vi "GoalieNormal.vi"(7 "AI Parameters":T1={"GotoKick"={"Dist do cone a frente"=0.0, "attacker farback"=1000.0, "Perto"=300.0, "min dist to kick"=0.0, "kick eps"=110.0, "Time to transition"=0.05}, "Attacker"={"CC chute"=0.09, "CC passe"=0.045, "Kick Force"=200.0, "D ball-robot Kick"=200.0, "D ball-robot Pass"=0.0}, "Defender"={"D max"=1700.0, "Vel p/ robô av"=1000.0, "Kick Force"=100.0, "D atk-def"=300.0, "D farback"=400.0}, "Timeout"={"Field/v in x"=6.0, "Dist Robots"=300, "Dist up in y"=300}, "Pose Striker"={"dist"=200.0, "Numeric"=-4.0, "dist 2"=200.0}, "Dist Stop"=300.0, "Distance when ball out"=200, "D central gap "=150.0} {"D central gap" format="%#_13g"; "Dist Stop" format="%#_13g"; "Pose Striker"."Numeric" format="%#_13g"; "Defender"."Kick Force" format="%#_13g"; "Defender"."Vel p/ robô av" format="%#_13g"; "Attacker"."D ball-robot Kick" format="%#_13g"; "Attacker"."Kick Force" format="%#_13g"; "Attacker"."CC passe" format="%#_13g"; "Attacker"."CC chute" format="%#_13g"; "GotoKick"."min dist to kick" format="%#_13g"; "GotoKick"."Perto" format="%#_13g"; "GotoKick"."attacker farback" format="%#_13g"; "GotoKick"."Dist do cone a frente" format="%#_13g"}, 8 "Robot":T2={"id"=0, "function"=enum."Attacker", "x"=0.0, "y"=0.0, "orientation"=0.0, "v_tangent"=0.0, "v_normal"=0.0, "v_ang"=0.0, "kick_x"=0.0, "kick_z"=0.0, "dribble"=FALSE, "Timestamp"=timestamp(0 s since 1904-01-01), "dest_x"=0.0, "dest_y"=0.0, "dest_orientation"=0.0, "estimatives"={"est_v_tangent"=0.0, "est_v_normal"=0.0, "est_vx"=0.0, "est_vy"=0.0, "Pos Robot Est"=[]}, "dest_x_kick"=0.0, "dest_y_kick"=0.0, "Gap Coord"=[], "States"=enum."GoToTangent"}, 10 "Field defense":dbl[](array[numeric]), 11 "IA Input":T5={"our_robots"=[], "enemy_robots"=[], "balls"=[], "geometry"={"line_width"=0, "field_length"=0, "field_width"=0, "boundary_width"=0, "referee_width"=0, "goal_width"=0, "goal_depth"=0, "goal_wall_width"=0, "center_circle_radius"=0, "defense_radius"=0, "defense_stretch"=0, "free_kick_from_defense_dist"=0, "penalty_spot_from_field_line_dist"=0, "penalty_line_from_spot_dist"=0}, "IA Judge"={"stage"="", "command"="", "our_goalie_id"=0.0, "enemy_goalie_id"=0.0, "command enum"=enum."Halt", "Time"=enum."Azul"}, "Received Timestamp"=timestamp(0 s since 1904-01-01), "Events"={"Touch"=FALSE, "Ball out"=FALSE, "id touch"=0.0, "Ball out of \nVision"=FALSE, "Ball inside \nGoalie area"=FALSE, "Robot not responding"=FALSE, "Robots responding status"=[1.0, 1.0, 1.0, 1.0, 1.0, 1.0], "Enemy Ball \nPossession"=FALSE, "Pass State"=FALSE, "id end of pass"=0.0, "Kick"=FALSE, "Id Possession"=0.0}}) -> (2 "output cluster":T2={"id"=0, "function"=enum."Attacker", "x"=0.0, "y"=0.0, "orientation"=0.0, "v_tangent"=0.0, "v_normal"=0.0, "v_ang"=0.0, "kick_x"=0.0, "kick_z"=0.0, "dribble"=FALSE, "Timestamp"=timestamp(0 s since 1904-01-01), "dest_x"=0.0, "dest_y"=0.0, "dest_orientation"=0.0, "estimatives"={"est_v_tangent"=0.0, "est_v_normal"=0.0, "est_vx"=0.0, "est_vy"=0.0, "Pos Robot Est"=[]}, "dest_x_kick"=0.0, "dest_y_kick"=0.0, "Gap Coord"=[], "States"=enum."GoToTangent"})   [LabVIEW 2016]
uses:
  Core/AI Input.ctl
  Core/AI Robot.ctl
  Functions Enum.ctl
  AttackerStates.ctl
  Core/AI Ball.ctl
  Core/Field Size.ctl
  Core/AI Judge.ctl
  Command Enum.ctl
  Util/Events/Events.ctl
  AI Parameters.ctl
panel:
  in  "Time kick (s)":dbl=1.0 caption="Time Target (s)"
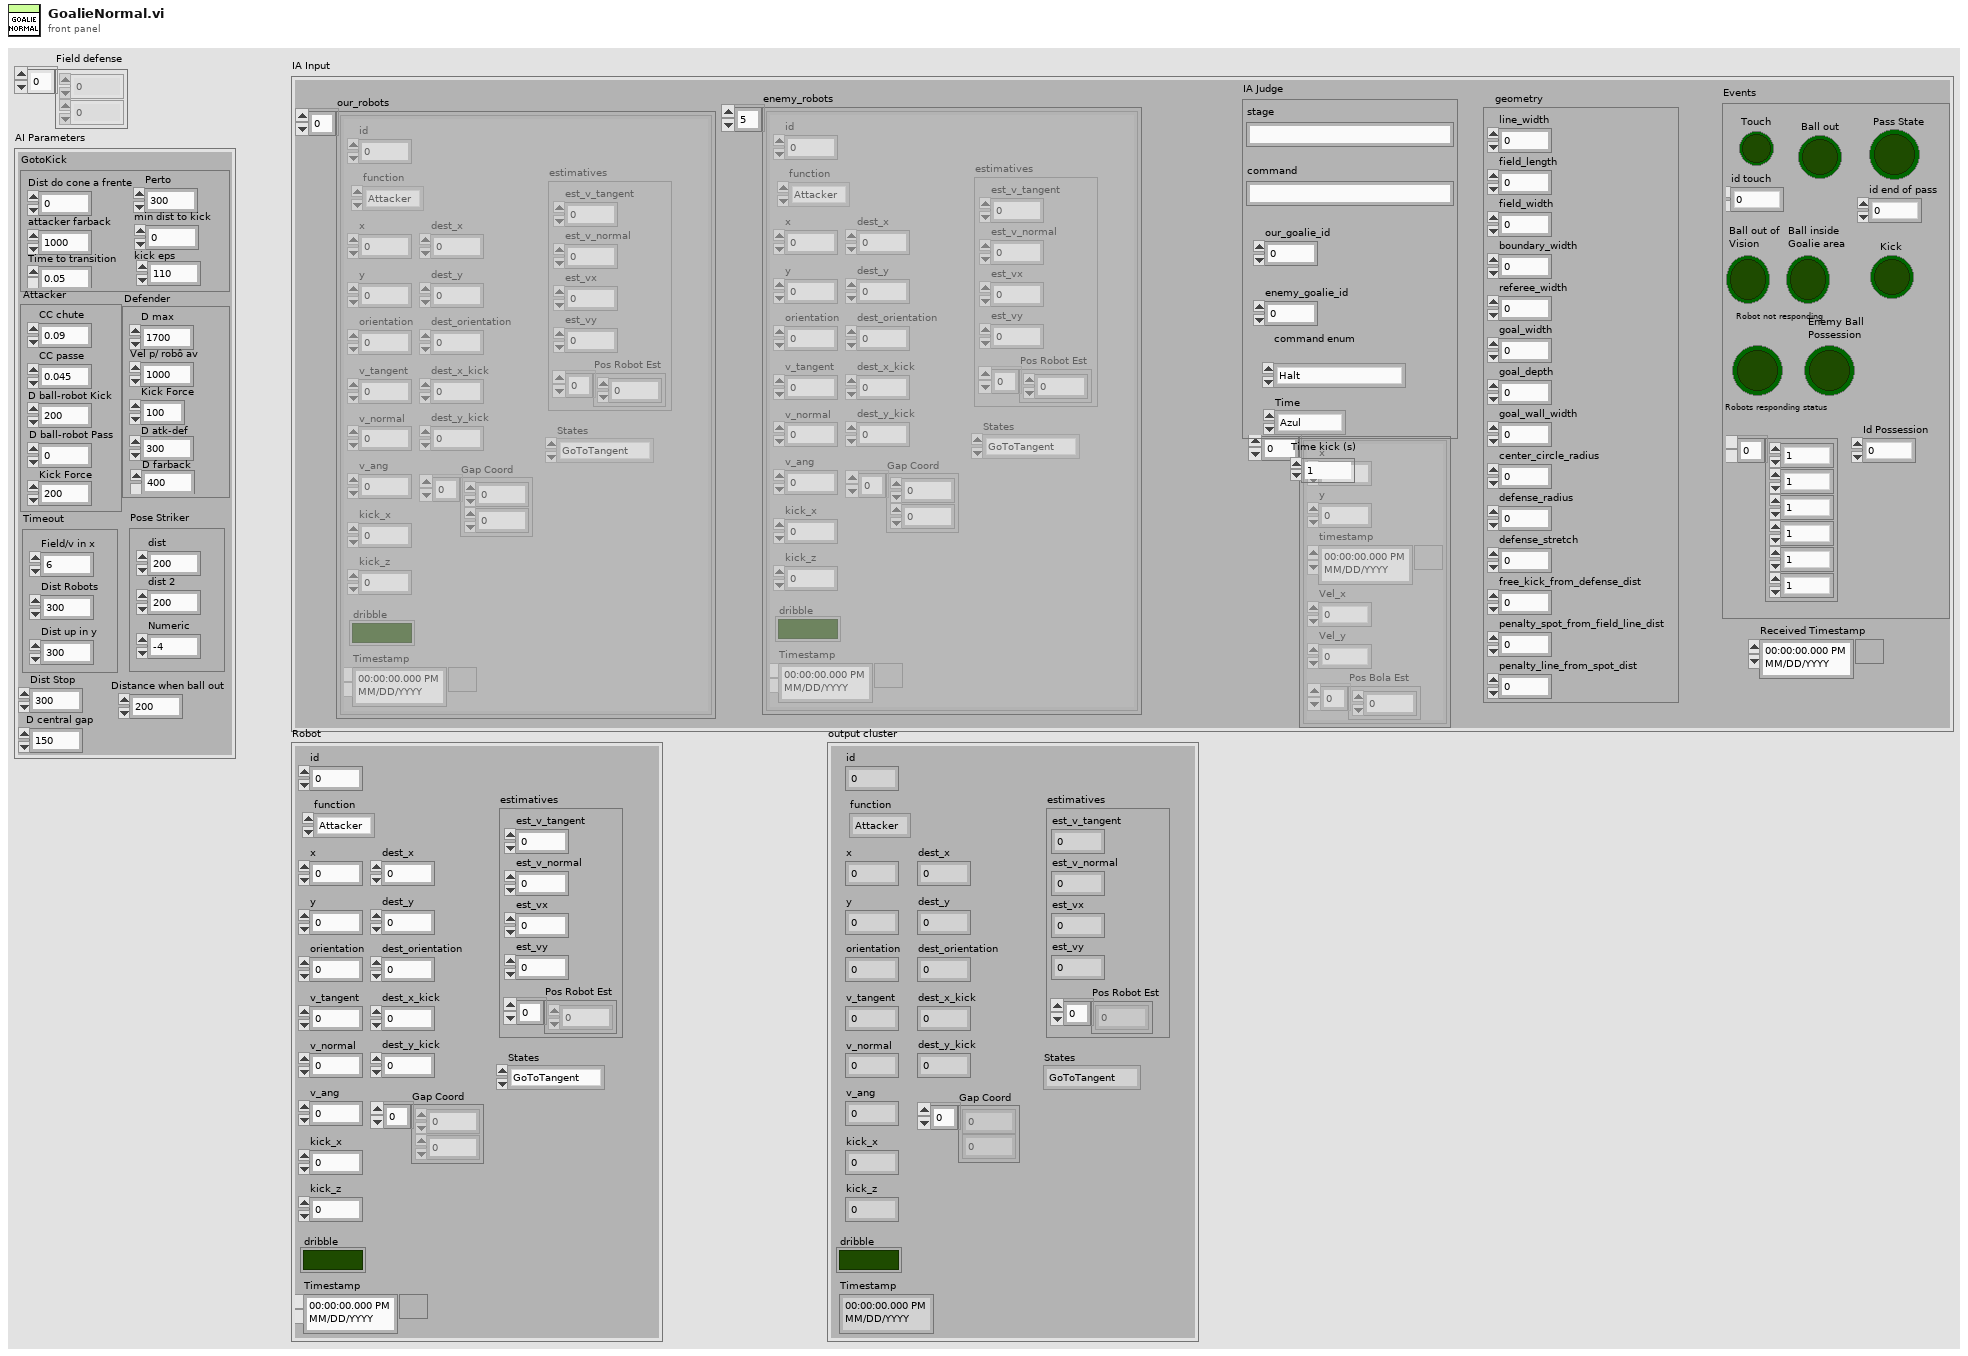
[diagram p1: front panel]
types:
  T1 = typedef "AI Parameters.ctl" = cluster{"GotoKick":cluster{"Dist do cone a frente":dbl, "attacker farback":dbl, "Perto":dbl, "min dist to kick":dbl, "kick eps":dbl, "Time to transition":dbl}, "Attacker":cluster{"CC chute":dbl, "CC passe":dbl, "Kick Force":dbl, "D ball-robot Kick":dbl, "D ball-robot Pass":dbl}, "Defender":cluster{"D max":dbl, "Vel p/ robô av":dbl, "Kick Force":dbl, "D atk-def":dbl, "D farback":dbl}, "Timeout":cluster{"Field/v in x":dbl, "Dist Robots":u32, "Dist up in y":u32}, "Pose Striker":cluster{"dist":dbl, "Numeric":dbl, "dist 2":dbl}, "Dist Stop":dbl, "Distance when ball out":i32, "D central gap ":dbl}
  T2 = typedef "AI Robot.ctl" = cluster{"id":u32, "function":T3, "x":dbl, "y":dbl, "orientation":dbl, "v_tangent":dbl, "v_normal":dbl, "v_ang":dbl, "kick_x":dbl, "kick_z":dbl, "dribble":bool, "Timestamp":timestamp, "dest_x":dbl, "dest_y":dbl, "dest_orientation":dbl, "estimatives":cluster{"est_v_tangent":dbl, "est_v_normal":dbl, "est_vx":dbl, "est_vy":dbl, "Pos Robot Est":dbl[]}, "dest_x_kick":dbl, "dest_y_kick":dbl, "Gap Coord":dbl[], "States":T4}
  T3 = typedef "Functions Enum.ctl" = enum16{"Attacker", "Goalie", "Defender", "Striker", "Goto 0", "Dummy", "Kicker", "ZigZag"}
  T4 = typedef "AttackerStates.ctl" = enum16{"Pass", "GoToTangent", "BallGetting", "GoToKick", ""}
  T5 = typedef "AI Input.ctl" = cluster{"our_robots":T2[], "enemy_robots":T2[], "balls":T6[], "geometry":T7, "IA Judge":T8, "Received Timestamp":timestamp, "Events":T10}
  T6 = typedef "AI Ball.ctl" = cluster{"x":dbl, "y":dbl, "timestamp":timestamp, "Vel_x":dbl, "Vel_y":dbl, "Pos Bola Est":dbl[]}
  T7 = typedef "Field Size.ctl" = cluster{"line_width":u32, "field_length":u32, "field_width":u32, "boundary_width":u32, "referee_width":u32, "goal_width":u32, "goal_depth":u32, "goal_wall_width":u32, "center_circle_radius":u32, "defense_radius":u32, "defense_stretch":u32, "free_kick_from_defense_dist":u32, "penalty_spot_from_field_line_dist":u32, "penalty_line_from_spot_dist":u32}
  T8 = typedef "AI Judge.ctl" = cluster{"stage":string, "command":string, "our_goalie_id":dbl, "enemy_goalie_id":dbl, "command enum":T9, "Time":enum16{"Azul", "Amarelo"}}
  T9 = typedef "Command Enum.ctl" = enum16{"Halt", "Stop", "Force Start", "PKA Normal Start", "Prepare Kickoff Ally", "PKE Normal Start", "Prepare Kickoff Enemy", "Prepare Penalty Ally", "PPA Normal Start", "Prepare Penalty Enemy", "PPE Normal Start", "Direct Free Enemy", "Direct Free Ally", "Indirect Free Enemy", "Indirect Free Ally", "Timeout Enemy", "Timeout Ally", "Goal Enemy", "Goal Ally", "Ball Placement Enemy", "Ball Placement Ally", "Normal Half Time", "Extra Time Break", "Extra Half Time", "None"}
  T10 = typedef "Events.ctl" = cluster{"Touch":bool, "Ball out":bool, "id touch":dbl, "Ball out of \nVision":bool, "Ball inside \nGoalie area":bool, "Robot not responding":bool, "Robots responding status":dbl[], "Enemy Ball \nPossession":bool, "Pass State":bool, "id end of pass":dbl, "Kick":bool, "Id Possession":dbl}
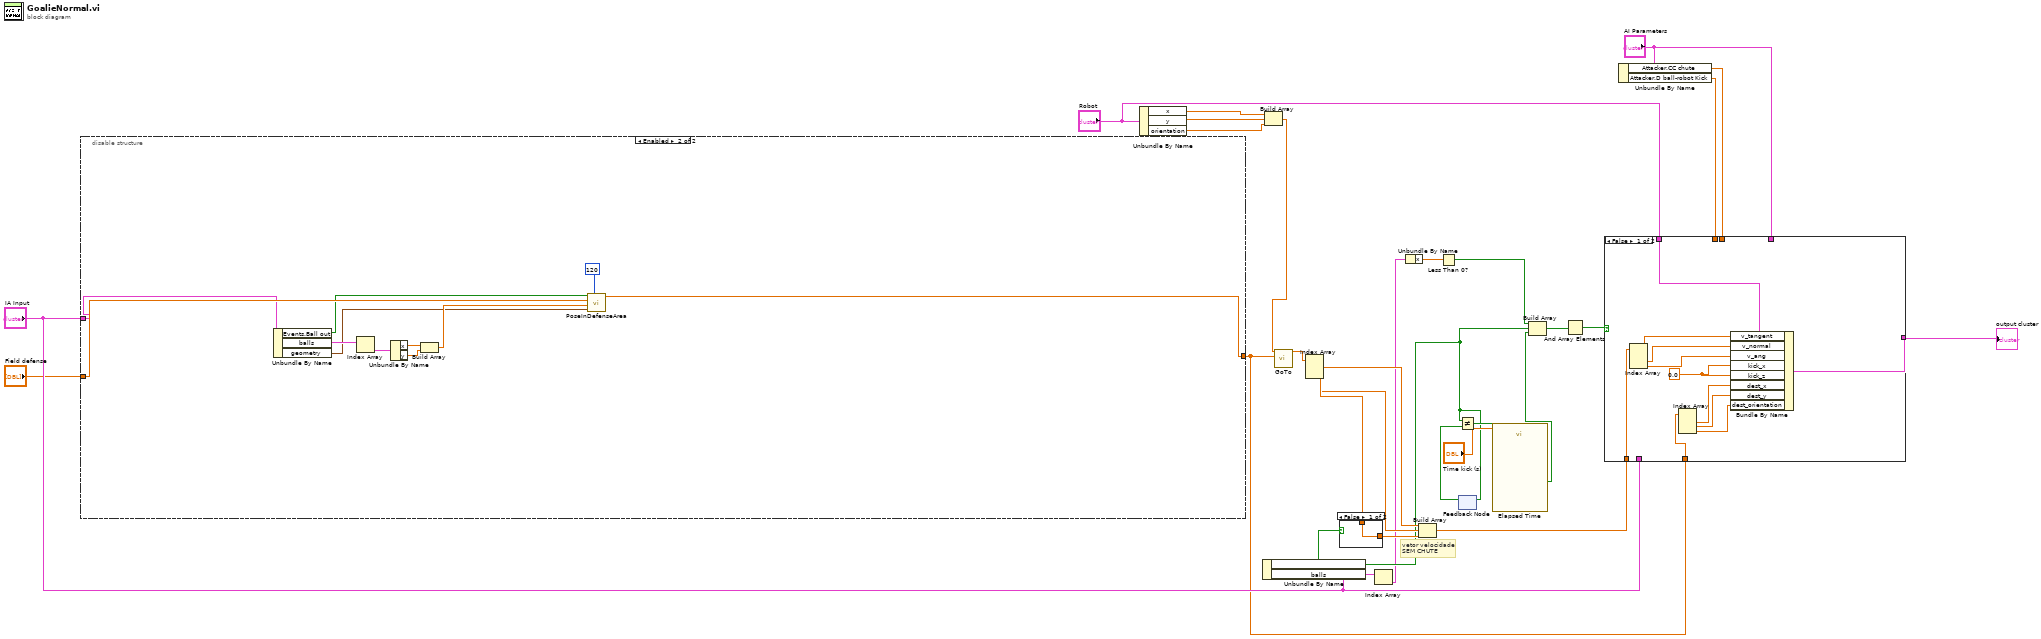
[diagram p0: block diagram]
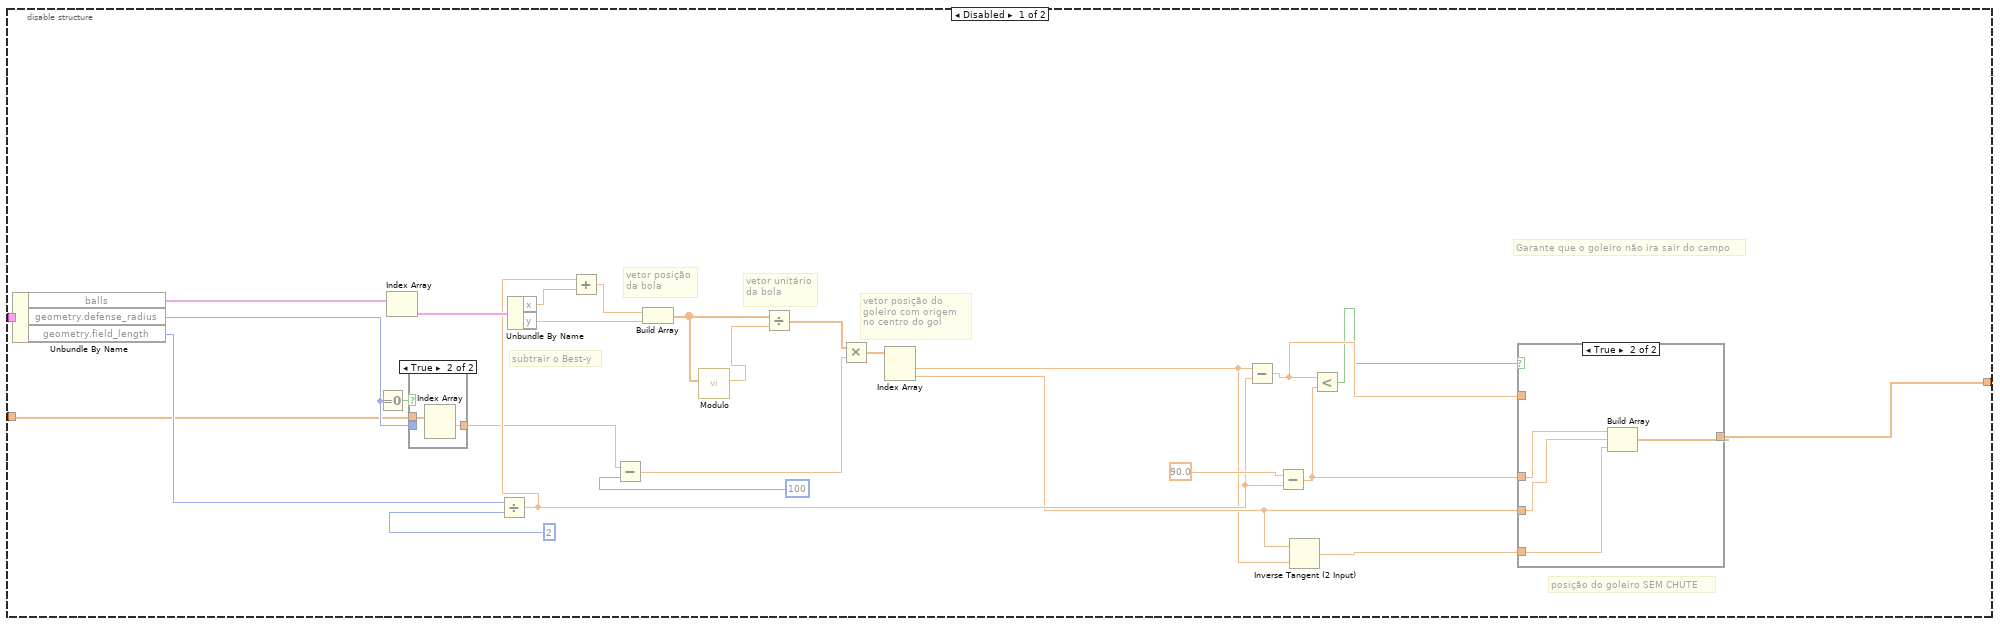
[diagram p2: hidden frame]
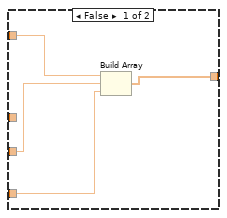
[diagram p4: hidden frame]
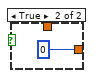
[diagram p5: hidden frame]
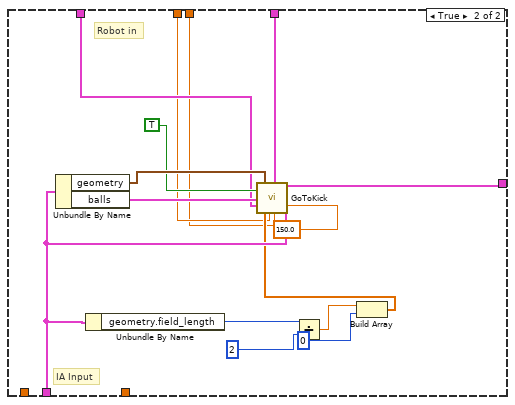
[diagram p6: hidden frame]
diagram:
  # "vetor velocidade SEM CHUTE"
  n1 = disable-structure shown="Enabled" {
    disable-tunnel: "IA Input" -> [w35 w72]
    disable-tunnel: [w34 w78] -> w5
    disable-tunnel: "Field defense" -> [w30 w77]
    frame Disabled {
      # "posição do goleiro SEM CHUTE"
      # "Garante que o goleiro não ira sair do campo"
      # "vetor posição do goleiro com origem no centro do gol"
      # "subtrair o Best-y"
      # "vetor unitário da bola"
      # "vetor posição da bola"
      n2 = Unbundle By Name(w35) -> ("balls"=w56:T6[], "geometry.defense_radius"=w31:u32, "geometry.field_length"=w41:u32)
      n3 = Equal To 0?(x=w31) -> (x = 0?=w32:bool)
      n4 = Index Array(array=w56) -> (element=w55:T6)  [unwired: 1 in]
      n5 = case shown="True" w32 {
        tunnel: [w57 w58] -> w33
        tunnel: w31 -> [w57 _]
        tunnel: w30 -> [_ w59]
        frame False {
        }
        frame True {
          n6 = Index Array(array=w59) -> (element #2=w58:dbl)  [unwired: 2 in, 1 out]
        }
      }
      n7 = Divide(x=w41, y=u32 2) -> (x/y=w40:dbl)
      n8 = Unbundle By Name(w55) -> ("x"=w42:dbl, "y"=w43:dbl)
      n9 = Add(x=w40, y=w42) -> (x+y=w39:dbl)
      n10 = Subtract(x=w33, y=u32 100) -> (x-y=w51:dbl)
      n11 = Build Array(w39, w43) -> (w54:dbl[])
      n12 = call "Modulo.vi"("2D vector"=w54) -> ("Modulo"=w53:dbl)  [unwired: 10 in]
      n13 = Divide(x=w54, y=w53) -> (x/y=w52:dbl[])
      n14 = Multiply(x=w52, y=w51) -> (x*y=w49:dbl[])
      n15 = Index Array(array=w49) -> (element #1=w37:dbl, element #2=w38:dbl)  [unwired: 2 in]
      n16 = Subtract(x=w37, y=w40) -> (x-y=w45:dbl)
      n17 = Subtract(x=90.0, y=w40) -> (x-y=w46:dbl)
      n18 = Inverse Tangent (2 Input)(1:w37, 2:w38) -> (0:w36:dbl)
      n19 = Less?(x=w45, y=w46) -> (x < y?=w44:bool)
      n20 = case shown="True" w44 {
        tunnel: w38 -> [w62 w65]
        tunnel: w46 -> [_ w67]
        tunnel: w45 -> [w63 _]
        tunnel: [w61 w66] -> w34
        tunnel: w36 -> [w60 w64]
        frame False {
          n21 = Build Array(w63, w62, w60) -> (w61:dbl[])
        }
        frame True {
          n22 = Build Array(w67, w65, w64) -> (w66:dbl[])
        }
      }
    }
    frame Enabled {
      n23 = Unbundle By Name(w72) -> ("Events.Ball out"=w68:bool, "balls"=w71:T6[], "geometry"=w69:T7)
      n24 = Index Array(array=w71) -> (element=w73:T6)  [unwired: 1 in]
      n25 = Unbundle By Name(w73) -> ("x"=w74:dbl, "y"=w75:dbl)
      n26 = Build Array(w74, w75) -> (w70:dbl[])
      n27 = call "PoseInDefenseArea.vi"("Recuo"=u32 120, "geometry"=w69, "Ball"=w70, "Field defense"=w77, "Events.Ball out"=w68) -> ("Array"=w78:dbl[])  [unwired: 6 in]
    }
  }
  n28 = Unbundle By Name("Robot") -> ("x"=w29:dbl, "y"=w28:dbl, "orientation"=w27:dbl)
  n29 = Unbundle By Name("IA Input") -> ("Events.Ball inside \nGoalie area"=w12:bool, "balls"=w9:T6[])
  n30 = Build Array(w29, w28, w27) -> (w26:dbl[])
  n31 = call "GoTo.vi"("Target"=w5, "Position"=w26) -> ("Output\nVelocity"=w25:dbl[])  [unwired: 8 in, 1 out]
  n32 = Index Array(array=w25) -> (element #1=w19:dbl, element #2=w20:dbl, element #3=w21:dbl)  [unwired: 3 in]
  n33 = case shown="False" w12 {
    tunnel: [w79 0] -> w22
    tunnel: w21 -> [w79 _]
    frame False {
    }
    frame True {
    }
  }
  n34 = Index Array(array=w9) -> (element=w8:T6)  [unwired: 1 in]
  n35 = Unbundle By Name(w8) -> ("x"=w7:dbl)
  n36 = Build Array(w19, w20, w22) -> (w17:dbl[])
  n37 = Less Than 0?(x=w7) -> (x < 0?=w6:bool)
  n38 = feedback #1() -> (w13:bool)  [unwired: 1 in]
  n39 = feedback-in #1(w12) -> ()
  n40 = Not Equal?(x=w12, y=w13) -> (x != y?=w15:bool)
  n41 = call "Elapsed Time"("Time Target (s)"="Time kick (s)", "Reset"=w15) -> ("Time has Elapsed"=w14:bool)  [unwired: 10 in, 7 out]
  n42 = Build Array(w6, w12, w14) -> (w10:bool[])
  n43 = And Array Elements(Boolean array=w10) -> (logical AND=w11:bool)
  n44 = Unbundle By Name("AI Parameters") -> ("Attacker.CC chute"=w2:dbl, "Attacker.D ball-robot Kick"=w3:dbl)
  n45 = case shown="False" w11 {
    tunnel: "IA Input" -> [_ w100]
    tunnel: "Robot" -> [w91 w103]
    tunnel: [w90 w102] -> w18
    tunnel: w17 -> [w88 _]
    tunnel: w5 -> [w84 _]
    tunnel: "AI Parameters" -> [_ w94]
    tunnel: w3 -> [_ w93]
    tunnel: w2 -> [_ w92]
    frame False {
      w89 = 0.0 ("kick_z")
      n46 = Index Array(array=w88) -> (element #1=w87:dbl, element #2=w86:dbl, element #3=w85:dbl)  [unwired: 3 in]
      n47 = Index Array(array=w84) -> (element #1=w83:dbl, element #2=w82:dbl, element #3=w81:dbl)  [unwired: 3 in]
      n48 = Bundle By Name(cluster=w91, "v_tangent"=w87, "v_normal"=w86, "v_ang"=w85, "kick_x"=w89, "kick_z"=w89, "dest_x"=w83, "dest_y"=w82, "dest_orientation"=w81) -> (w90:T2)
    }
    frame True {
      # "Robot in"
      # "IA Input"
      n49 = Unbundle By Name(w100) -> ("geometry"=w106:T7, "balls"=w105:T6[])
      n50 = Unbundle By Name(w100) -> ("geometry.field_length"=w99:u32)
      n51 = Divide(x=w99, y=u32 2) -> (x/y=w97:dbl)
      n52 = Build Array(w97, 0) -> (w95:dbl[])
      n53 = call "GoToKick.vi"("goleiro?"=TRUE, "balls"=w105, "Robot in in"=w103, "Field Size in"=w106, "Target"=w95, "D ball - robot"=w93, "AI Parameters"=w94, "Cone de chute"=w92, "Kick Force"=150.0, "IA State Input in"=w100) -> ("Robot out"=w102:T2)  [unwired: 6 in, 3 out]
    }
  }
  "output cluster" <- w18
